vi "DB Update Data(Feedback_nc).vi"(0 "Connncet State":T1, 1 "data":variant, 2 "Updaate":string, 3 "Sel":string, 5 "table":string, 9 "Code":string, 11 "error in (no error)":errorcluster caption="错误输入（无错误）", 12 "Sel index":i32, 13 "Pos":cluster{"index":i32, "Len":i32}) -> (4 "Connncet State out":T1, 6 "State":bool, 15 "error out":errorcluster caption="错误输出")   [LabVIEW 2014]
uses:
  <vilib>/addons/database/NI_Database_API.lvlib
  Ctr/Constr.ctl
  <vilib>/addons/database/Connection.llb/Conn ObjectReference.ctl
  Ctr/Conneect State.ctl
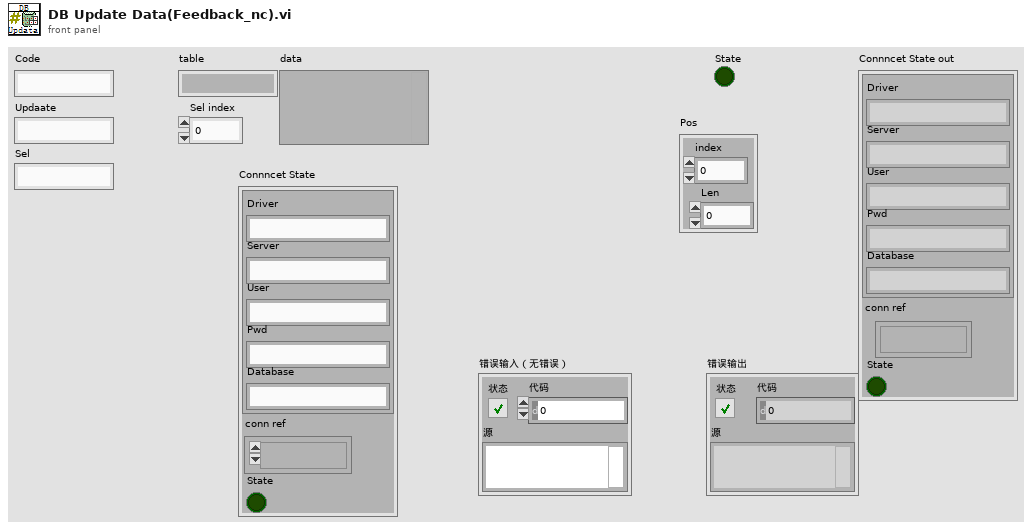
[diagram p1: front panel]
types:
  T1 = typedef "Conneect State.ctl" = cluster{"Constr":T2, "conn ref":T3, "State":bool}
  T2 = typedef "Constr.ctl" = cluster{"Driver":string, "Server":string, "User":string, "Pwd":string, "Database":string}
  T3 = typedef "NI_Database_API.lvlib/Conn ObjectReference.ctl" = refnum<k1>
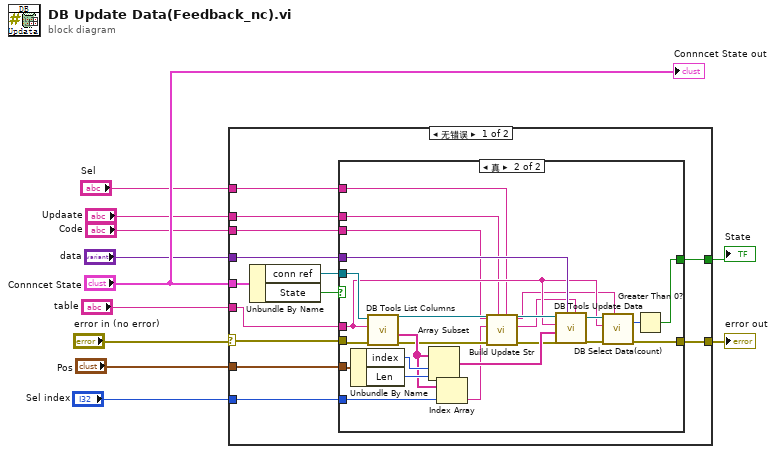
[diagram p0: block diagram]
diagram:
  n1 = case shown="无错误" "error in (no error)" {
    selector: "error in (no error)" -> [w23 w50]
    tunnel: "Connncet State" -> [w24 _]
    tunnel: "table" -> [w20 _]
    tunnel: "data" -> [w19 _]
    tunnel: "Pos" -> [w18 _]
    tunnel: "Sel index" -> [w17 _]
    tunnel: [w16 w50] -> w5
    tunnel: [w15 _] -> w4
    tunnel: "Code" -> [w14 _]
    tunnel: "Updaate" -> [w13 _]
    tunnel: "Sel" -> [w12 _]
    frame No Error {
      n2 = Unbundle By Name(w24) -> ("conn ref"=w21:T3, "State"=w22:bool)
      n3 = case shown="真" w22 {
        tunnel: w23 -> [w25 w49]
        tunnel: w21 -> [_ w48]
        tunnel: w20 -> [_ w39]
        tunnel: w19 -> [_ w46]
        tunnel: w18 -> [_ w44]
        tunnel: w17 -> [_ w37]
        tunnel: [w25 w36] -> w16
        tunnel: [_ w34] -> w15
        tunnel: w14 -> [_ w32]
        tunnel: w13 -> [_ w30]
        tunnel: w12 -> [_ w29]
        frame False {
        }
        frame True {
          n4 = Unbundle By Name(w44) -> ("index"=w43:i32, "Len"=w42:i32)
          n5 = call <vilib>:"DB Tools List Columns.vi"("error in (no error)"=w49, "table"=w39, "connection reference"=w48) -> ("error out"=w33:errorcluster, "columns"=w38:string[], "connection reference out"=w47:T3)  [unwired: 1 in, 1 out]
          n6 = Array Subset(array=w38, index=w43, length=w42) -> (w45:string[])
          n7 = Index Array(array=w38, index=w37) -> (element=w31:string)
          n8 = call "Build Update Str.vi"("sel"=w29, "update"=w30, "error in (no error)"=w33, "Col"=w31, "code"=w32) -> ("error out"=w28:errorcluster, "Update"=w26:string, "Sel"=w27:string)  [unwired: 4 in]
          n9 = call <vilib>:"DB Tools Update Data.vi"("condition"=w26, "data"=w46, "error in (no error)"=w28, "columns"=w45, "table"=w39, "connection reference"=w47) -> ("error out"=w41:errorcluster, "connection reference out"=w40:T3)  [unwired: 4 in]
          n10 = call "DB Select Data(count).vi"("condition"=w27, "error in (no error)"=w41, "table"=w39, "connection reference"=w40) -> ("error out"=w36:errorcluster, "Count"=w35:i32)  [unwired: 5 in, 1 out]
          n11 = Greater Than 0?(x=w35) -> (x > 0?=w34:bool)
        }
      }
    }
    frame Error {
    }
  }
  "error out" <- w5
  "State" <- w4
  "Connncet State out" <- "Connncet State"
